vi "Ctor.vi"(5 "Blank Type (Built-In)":refnum<class "ArrayBlank.lvclass">, 6 "Panel Borders? (T)":bool=TRUE, 7 "Dynamic Sizing? (F)":bool, 8 "error in (no error)":errorcluster, 9 "Scrollbar":refnum<vi>, 10 "SubPanels":refnum<vi>[](array[refnum])) -> (0 "error out":errorcluster, 3 "PanelArray out":refnum<class "PanelArray.lvclass">)   [LabVIEW 2018, in "OOPanel.lvlib" / "PanelArray.lvclass"]
uses:
  PanelArray.lvclass
  ArrayBlank/ArrayBlank.lvclass
  Ref Data.ctl
  State.ctl
  Refs.ctl
  Events.ctl
  Scrolling.ctl
  Panels.ctl
  Panel/Panel.lvclass
  PanelArray.lvclass/PanelArray.ctl
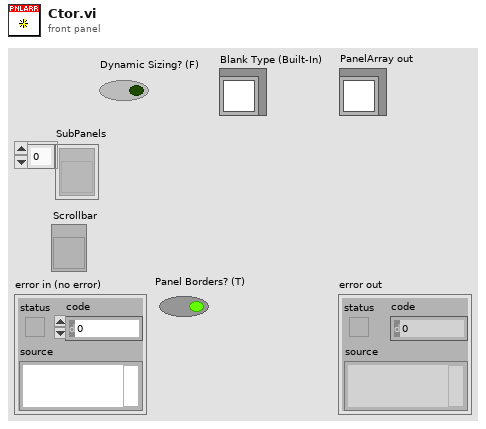
[diagram p1: front panel]
types:
  T1 = typedef "OOPanel.lvlib/PanelArray.lvclass/Ref Data.ctl" = cluster{"State":T2, "Refs":T3, "Events":T4, "Scrolling":T5, "Panels":T6}
  T2 = typedef "OOPanel.lvlib/PanelArray.lvclass/State.ctl" = cluster{"Defer Updates":bool, "Running":bool, "Dynamic Sizing":bool, "Borders":bool}
  T3 = typedef "OOPanel.lvlib/PanelArray.lvclass/Refs.ctl" = cluster{"SubPanels":refnum<vi>[], "Scrollbar":refnum<vi>, "Owning Panel":refnum<vi>}
  T4 = typedef "OOPanel.lvlib/PanelArray.lvclass/Events.ctl" = cluster{"Close":refnum<user-event>}
  T5 = typedef "OOPanel.lvlib/PanelArray.lvclass/Scrolling.ctl" = cluster{"Size":i32, "Max":i32, "Current":i32, "Top Index":i32, "Heights":i32[]}
  T6 = typedef "OOPanel.lvlib/PanelArray.lvclass/Panels.ctl" = cluster{"All":refnum<class "Panel.lvclass">[], "Visible":refnum<class "Panel.lvclass">[], "Blank":refnum<class "ArrayBlank.lvclass">}
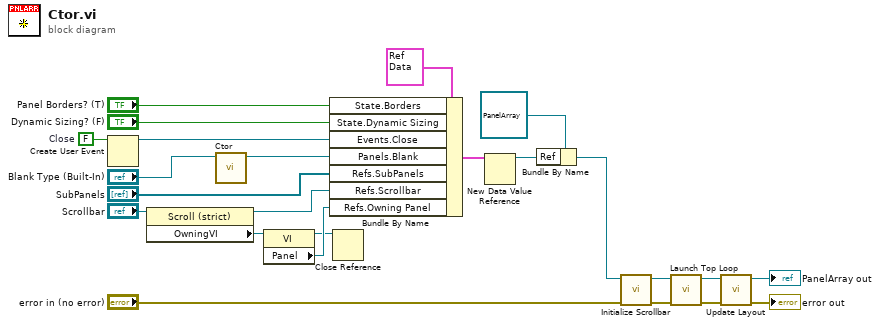
[diagram p0: block diagram]
diagram:
  w20 = FALSE  # Close
  n1 = Create User Event(user event datatype=w20) -> (user event=w19:refnum<user-event>)  [unwired: 1 in, 1 out]
  n2 = property class="Scroll (strict)"(reference="Scrollbar") -> (reference out=w8:refnum<vi>, "OwningVI"=w18:refnum<vi>)  [unwired: 1 in, 1 out]
  n3 = call-dynamic "Ctor.vi"("ArrayBlank in"="Blank Type (Built-In)") -> ("ArrayBlank out"=w13:refnum<class "ArrayBlank.lvclass">)  [unwired: 9 in, 1 out]
  n4 = property class="VI"(reference=w18) -> (reference out=w16:refnum<vi>, "Panel"=w17:refnum<vi>)  [unwired: 1 in, 1 out]
  n5 = Bundle By Name(cluster=T1 {"State"={"Defer Updates"=FALSE, "Running"=FALSE, "Dynamic Sizing"=FALSE, "Borders"=FALSE}, "Refs"={"SubPanels"=[], "Scrollbar"=refnum, "Owning Panel"=refnum}, "Events"={"Close"=refnum}, "Scrolling"={"Size"=0, "Max"=0, "Current"=0, "Top Index"=0, "Heights"=[]}, "Panels"={"All"=[], "Visible"=[], "Blank"=refnum}} ("Ref Data"), "State.Borders"="Panel Borders? (T)", "State.Dynamic Sizing"="Dynamic Sizing? (F)", "Events.Close"=w19, "Panels.Blank"=w13, "Refs.SubPanels"="SubPanels", "Refs.Scrollbar"=w8, "Refs.Owning Panel"=w17) -> (w21:T1)
  n6 = Close Reference(reference=w16) -> ()  [unwired: 1 in, 1 out]
  n7 = New Data Value Reference(data value=w21) -> (data value reference=w24:refnum<data-value>)  [unwired: 1 in, 1 out]
  n8 = Bundle By Name(cluster=refnum<class "PanelArray.lvclass"> refnum ("PanelArray in"), "Ref"=w24) -> (w9:refnum<class "PanelArray.lvclass">)
  n9 = call "Initialize Scrollbar.vi"("error in (no error)"="error in (no error)", "PanelArray in"=w9) -> ("error out"=w11:errorcluster, "PanelArray out"=w10:refnum<class "PanelArray.lvclass">)  [unwired: 8 in]
  n10 = call "Launch Top Loop.vi"("error in (no error)"=w11, "PanelArray in"=w10) -> ("error out"=w3:errorcluster, "PanelArray out"=w4:refnum<class "PanelArray.lvclass">)  [unwired: 8 in]
  n11 = call "Update Layout.vi"("error in (no error)"=w3, "PanelArray in"=w4) -> ("error out"=→"error out":errorcluster, "PanelArray out"=→"PanelArray out":refnum<class "PanelArray.lvclass">)  [unwired: 8 in]
